vi "FS Body Functions.vi"(6 "Sketch/Body #":i32=1, 7 "Feature In":string="FeatureScript 1247;\nimport(path : \"onshape/std/geometry.fs\", version : \"1247.0\");\n\nannotation { \"Feature Type Name\" : \"LabVIEW Feature\" }\nexport const myFeature = defineFeature(function(context is Context, id is Id, definition is map)\n    precondition\n    {\n        // Define the parameters of the feature type\n    }\n    {\n        // Define the function's action\n\nvar sketch1 = newSketch(context, id + \"sketch1\", {\n                \"sketchPlane\" : qCreatedBy(makeId(\"Top\"), EntityType.FACE)\n        });\n        // Create sketch entities here\n        skRectangle(sketch1, \"rectangle1\", {\n                \"firstCorner\" : vector(0, 0) * inch,\n                \"secondCorner\" : vector(3, 4) * inch\n        });\n        \n        skSolve(sketch1);\n    });", 8 "Elipsoid":T1={"Center"={"x"=5.0, "y"=0.0, "z"=0.0}, "Radii"={"x"=3.0, "y"=3.0, "z"=3.0}}, 9 "Cylinder":T2={"Point 1"={"x"=0.0, "y"=0.0, "z"=0.0}, "Point 2"={"x"=1.0, "y"=1.0, "z"=1.0}, "Radius"=1.0}, 10 "Cuboid":T3={"Point 1"={"x"=0.0, "y"=0.0, "z"=0.0}, "Point 2"={"x"=1.0, "y"=1.0, "z"=1.0}}, 11 "Body Shape":T4=enum."Elipsoid") -> (3 "Feature Out":string="FeatureScript 1247;\nimport(path : \"onshape/std/geometry.fs\", version : \"1247.0\");\n\nannotation { \"Feature Type Name\" : \"LVFeat1\" }\nexport const myFeature = defineFeature(function(context is Context, id is Id, definition is map)\n    precondition\n    {\n        // Define the parameters of the feature type\n    }\n    {\n        // Define the function's action\n       fEllipsoid(context, id + \"ellipsoid1\", {\n                \"center\" : vector(5, 0, 0) * inch,\n                \"radius\" : vector(3, 3, 3) * inch,\n        });\n\nvar sketch1 = newSketch(context, id + \"sketch1\", {\n                \"sketchPlane\" : qCreatedBy(makeId(\"Top\"), EntityType.FACE)\n        });\n        // Create sketch entities here\n        skRectangle(sketch1, \"rectangle1\", {\n                \"firstCorner\" : vector(0, 0) * inch,\n                \"secondCorner\" : vector(3, 4) * inch\n        });\n        \n        skSolve(sketch1);\n    });")   [LabVIEW 2019]
uses:
  Body Shapes.ctl
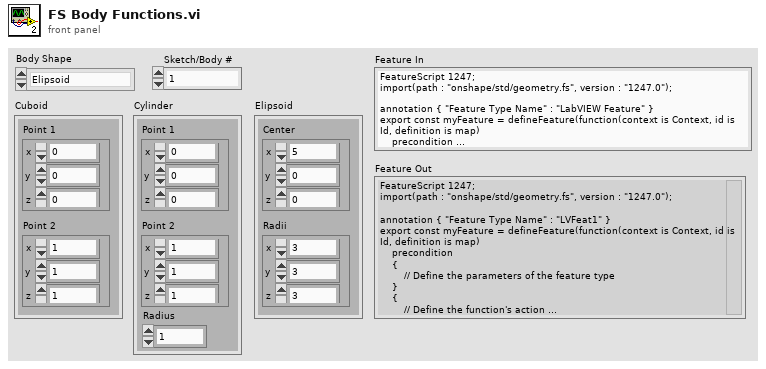
[diagram p1: front panel]
types:
  T1 = cluster{"Center":cluster{"x":dbl, "y":dbl, "z":dbl}, "Radii":cluster{"x":dbl, "y":dbl, "z":dbl}}
  T2 = cluster{"Point 1":cluster{"x":dbl, "y":dbl, "z":dbl}, "Point 2":cluster{"x":dbl, "y":dbl, "z":dbl}, "Radius":dbl}
  T3 = cluster{"Point 1":cluster{"x":dbl, "y":dbl, "z":dbl}, "Point 2":cluster{"x":dbl, "y":dbl, "z":dbl}}
  T4 = typedef "Body Shapes.ctl" = enum16{"Cuboid", "Cylinder", "Elipsoid"}
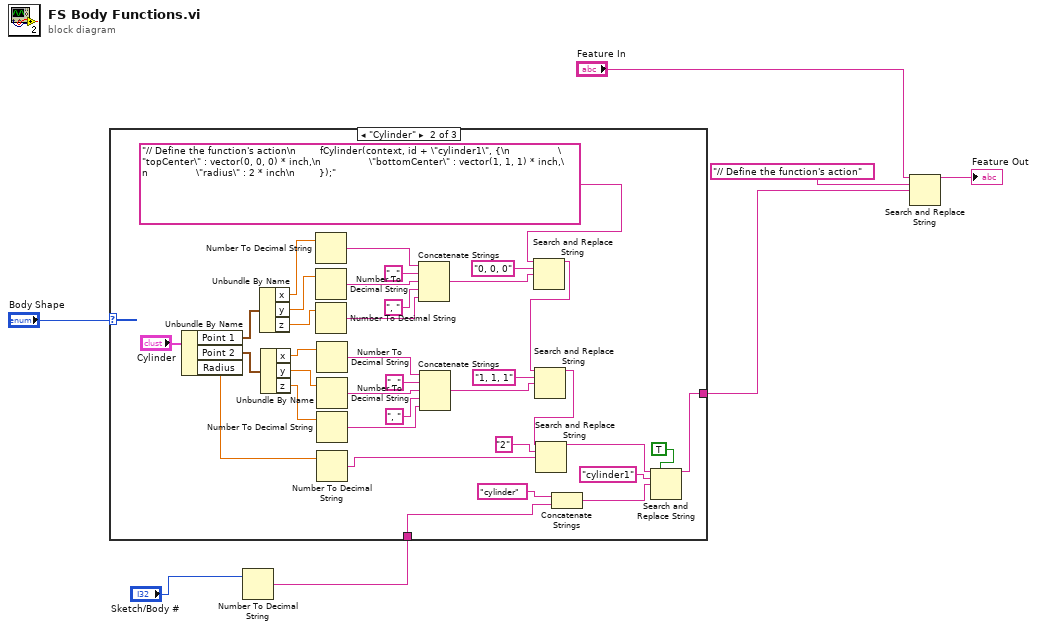
[diagram p0: block diagram]
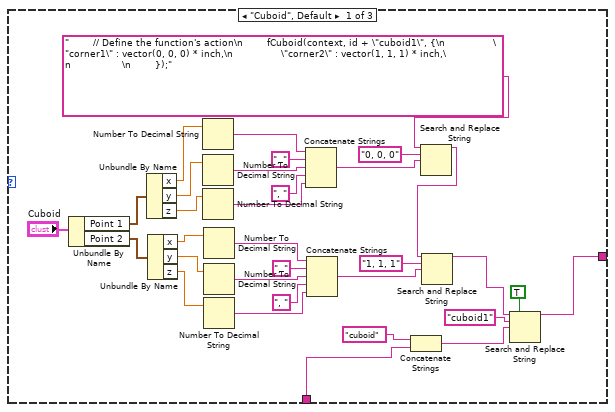
[diagram p2: hidden frame]
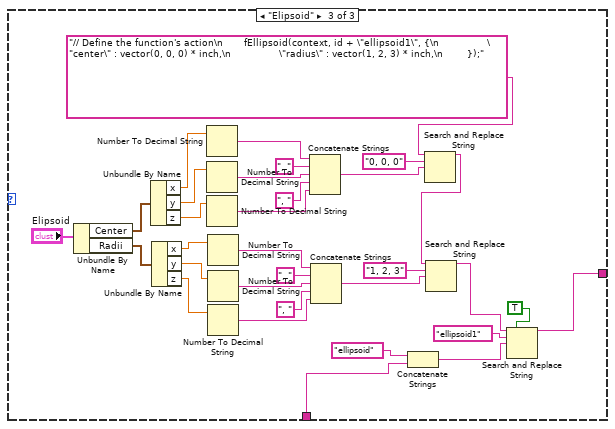
[diagram p3: hidden frame]
diagram:
  n1 = Number To Decimal String(number="Sketch/Body #") -> (decimal integer string=w1:string)  [unwired: 1 in]
  n2 = case shown="\"Cylinder\"" "Body Shape" {
    tunnel: [w8 w41 w76] -> w4
    tunnel: w1 -> [w10 w42 w78]
    frame "Cuboid", Default {
      n3 = Unbundle By Name("Cuboid") -> ("Point 1"=w37:cluster{"x":dbl, "y":dbl, "z":dbl}, "Point 2"=w36:cluster{"x":dbl, "y":dbl, "z":dbl})
      n4 = Unbundle By Name(w37) -> ("x"=w30:dbl, "y"=w29:dbl, "z"=w28:dbl)
      n5 = Unbundle By Name(w36) -> ("x"=w18:dbl, "y"=w17:dbl, "z"=w16:dbl)
      n6 = Number To Decimal String(number=w30) -> (decimal integer string=w34:string)  [unwired: 1 in]
      n7 = Number To Decimal String(number=w29) -> (decimal integer string=w33:string)  [unwired: 1 in]
      n8 = Number To Decimal String(number=w28) -> (decimal integer string=w31:string)  [unwired: 1 in]
      n9 = Number To Decimal String(number=w18) -> (decimal integer string=w21:string)  [unwired: 1 in]
      n10 = Number To Decimal String(number=w17) -> (decimal integer string=w22:string)  [unwired: 1 in]
      n11 = Number To Decimal String(number=w16) -> (decimal integer string=w24:string)  [unwired: 1 in]
      n12 = Concatenate Strings(w34, ", " ("regular expression"), w33, ", " ("regular expression"), w31) -> (w27:string)
      n13 = Concatenate Strings(w21, ", " ("regular expression"), w22, ", " ("regular expression"), w24) -> (w25:string)
      n14 = Concatenate Strings("cuboid" ("regular expression"), w10) -> (w11:string)
      n15 = Search and Replace String(input string="        // Define the function's action\n        fCuboid(context, id + \"cuboid1\", {\n                \"corner1\" : vector(0, 0, 0) * inch,\n                \"corner2\" : vector(1, 1, 1) * inch,\n                 \n        });" ("search string"), search string="0, 0, 0" ("regular expression"), replace string=w27) -> (result string=w15:string)  [unwired: 5 in, 3 out]
      n16 = Search and Replace String(input string=w15, search string="1, 1, 1" ("regular expression"), replace string=w25) -> (result string=w9:string)  [unwired: 5 in, 3 out]
      n17 = Search and Replace String(replace all?=TRUE ("replace all? (F)"), input string=w9, search string="cuboid1" ("regular expression"), replace string=w11) -> (result string=w8:string)  [unwired: 4 in, 3 out]
    }
    frame "Cylinder" {
      n18 = Unbundle By Name("Cylinder") -> ("Point 1"=w59:cluster{"x":dbl, "y":dbl, "z":dbl}, "Point 2"=w60:cluster{"x":dbl, "y":dbl, "z":dbl}, "Radius"=w50:dbl)
      n19 = Unbundle By Name(w59) -> ("x"=w64:dbl, "y"=w65:dbl, "z"=w66:dbl)
      n20 = Unbundle By Name(w60) -> ("x"=w72:dbl, "y"=w73:dbl, "z"=w74:dbl)
      n21 = Number To Decimal String(number=w64) -> (decimal integer string=w61:string)  [unwired: 1 in]
      n22 = Number To Decimal String(number=w65) -> (decimal integer string=w62:string)  [unwired: 1 in]
      n23 = Number To Decimal String(number=w66) -> (decimal integer string=w63:string)  [unwired: 1 in]
      n24 = Number To Decimal String(number=w72) -> (decimal integer string=w71:string)  [unwired: 1 in]
      n25 = Number To Decimal String(number=w73) -> (decimal integer string=w70:string)  [unwired: 1 in]
      n26 = Number To Decimal String(number=w74) -> (decimal integer string=w69:string)  [unwired: 1 in]
      n27 = Number To Decimal String(number=w50) -> (decimal integer string=w49:string)  [unwired: 1 in]
      n28 = Concatenate Strings(w61, ", " ("regular expression"), w62, ", " ("regular expression"), w63) -> (w67:string)
      n29 = Concatenate Strings(w71, ", " ("regular expression"), w70, ", " ("regular expression"), w69) -> (w68:string)
      n30 = Search and Replace String(input string="// Define the function's action\n        fCylinder(context, id + \"cylinder1\", {\n                \"topCenter\" : vector(0, 0, 0) * inch,\n                \"bottomCenter\" : vector(1, 1, 1) * inch,\n                \"radius\" : 2 * inch\n        });" ("search string"), search string="0, 0, 0" ("regular expression"), replace string=w67) -> (result string=w75:string)  [unwired: 5 in, 3 out]
      n31 = Search and Replace String(input string=w75, search string="1, 1, 1" ("regular expression"), replace string=w68) -> (result string=w47:string)  [unwired: 5 in, 3 out]
      n32 = Search and Replace String(input string=w47, search string="2" ("regular expression"), replace string=w49) -> (result string=w40:string)  [unwired: 5 in, 3 out]
      n33 = Concatenate Strings("cylinder" ("regular expression"), w42) -> (w46:string)
      n34 = Search and Replace String(replace all?=TRUE ("replace all? (F)"), input string=w40, search string="cylinder1" ("regular expression"), replace string=w46) -> (result string=w41:string)  [unwired: 4 in, 3 out]
    }
    frame "Elipsoid" {
      n35 = Unbundle By Name("Elipsoid") -> ("Center"=w105:cluster{"x":dbl, "y":dbl, "z":dbl}, "Radii"=w104:cluster{"x":dbl, "y":dbl, "z":dbl})
      n36 = Unbundle By Name(w105) -> ("x"=w98:dbl, "y"=w97:dbl, "z"=w96:dbl)
      n37 = Unbundle By Name(w104) -> ("x"=w86:dbl, "y"=w85:dbl, "z"=w84:dbl)
      n38 = Number To Decimal String(number=w98) -> (decimal integer string=w102:string)  [unwired: 1 in]
      n39 = Number To Decimal String(number=w97) -> (decimal integer string=w101:string)  [unwired: 1 in]
      n40 = Number To Decimal String(number=w96) -> (decimal integer string=w99:string)  [unwired: 1 in]
      n41 = Number To Decimal String(number=w86) -> (decimal integer string=w89:string)  [unwired: 1 in]
      n42 = Number To Decimal String(number=w85) -> (decimal integer string=w90:string)  [unwired: 1 in]
      n43 = Number To Decimal String(number=w84) -> (decimal integer string=w92:string)  [unwired: 1 in]
      n44 = Concatenate Strings(w102, ", " ("regular expression"), w101, ", " ("regular expression"), w99) -> (w95:string)
      n45 = Concatenate Strings(w89, ", " ("regular expression"), w90, ", " ("regular expression"), w92) -> (w93:string)
      n46 = Concatenate Strings("ellipsoid" ("regular expression"), w78) -> (w82:string)
      n47 = Search and Replace String(input string="// Define the function's action\n       fEllipsoid(context, id + \"ellipsoid1\", {\n                \"center\" : vector(0, 0, 0) * inch,\n                \"radius\" : vector(1, 2, 3) * inch,\n        });" ("search string"), search string="0, 0, 0" ("regular expression"), replace string=w95) -> (result string=w83:string)  [unwired: 5 in, 3 out]
      n48 = Search and Replace String(input string=w83, search string="1, 2, 3" ("regular expression"), replace string=w93) -> (result string=w77:string)  [unwired: 5 in, 3 out]
      n49 = Search and Replace String(replace all?=TRUE ("replace all? (F)"), input string=w77, search string="ellipsoid1" ("regular expression"), replace string=w82) -> (result string=w76:string)  [unwired: 4 in, 3 out]
    }
  }
  n50 = Search and Replace String(input string="Feature In", search string="// Define the function's action", replace string=w4) -> (result string=→"Feature Out":string)  [unwired: 5 in, 3 out]
